vi "DB_Deposit.vi"() -> ()   [LabVIEW 2013, in "ConfigDBLib.lvlib"]
uses:
  ConfigDBLib.lvlib
panel:
  in  "Deposited Amount":dbl
  in  "Account No":dbl
  out "Total Balance":dbl
  out "error out":errorcluster
  in  "error in (no error)":errorcluster
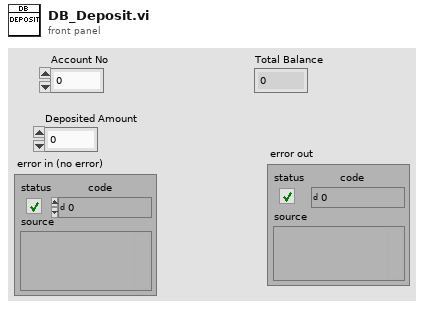
[diagram p1: front panel]
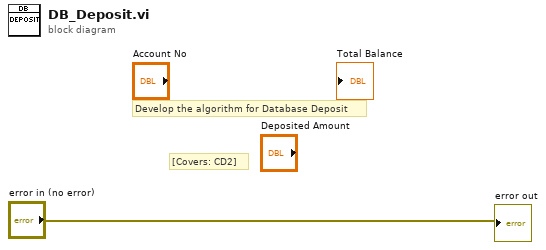
[diagram p0: block diagram]
diagram:
  # "[Covers: CD2]"
  # "Develop the algorithm for Database Deposit"
  "error out" <- "error in (no error)"
